vi "Open Sequence File.vi"(0 "Engine in":T3, 1 "Load Options (Default)":T2={"Use Search Dirs? (T)"=TRUE, "Conflict as Error? (T)"=TRUE, "Check Station Model? (F)"=FALSE, "Preload Modules? (T)"=TRUE, "Skip Load Callback? (F)"=FALSE, "Reload if Loaded? (F)"=FALSE}, 5 "File Path":path, 9 "Current Seq File (None)":T1, 11 "error in (no error)":errorcluster) -> (4 "Session Handle out":T3, 6 "SequenceFile":T1, 15 "error out":errorcluster)   [LabVIEW 2020, in "TSS.lvlib" / "Engine.lvclass"]
uses:
  Engine.lvclass
  Typedefs/Session Handle.ctl
  SequenceFile/Typedefs/Session Handle.ctl
  SequenceFile/SequenceFile.lvclass
  Data Types/File Load Options.ctl
  Open Sequence File Event Data.ctl
  Session Notification.ctl
  Engine.lvclass/Engine.ctl
  TSS.lvlib
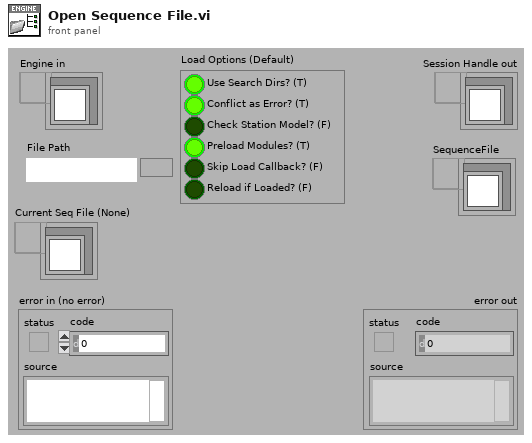
[diagram p1: front panel]
types:
  T1 = typedef "TSS.lvlib/SequenceFile.lvclass/Session Handle.ctl" = refnum<data-value>
  T2 = typedef "TSS.lvlib/File Load Options.ctl" = cluster{"Use Search Dirs? (T)":bool, "Conflict as Error? (T)":bool, "Check Station Model? (F)":bool, "Preload Modules? (T)":bool, "Skip Load Callback? (F)":bool, "Reload if Loaded? (F)":bool}
  T3 = typedef "TSS.lvlib/Engine.lvclass/Session Handle.ctl" = refnum<data-value>
  T4 = typedef "TSS.lvlib/Engine.lvclass/Session Notification.ctl" = cluster{"Session":refnum<data-value>, "Error":errorcluster}
  T5 = typedef "TSS.lvlib/Engine.lvclass/Open Sequence File Event Data.ctl" = cluster{"File Path":path, "Load Options":T2, "Current Seq File (None)":T1, "Session Notifier":refnum<notifier>, "Engine":refnum<data-value>}
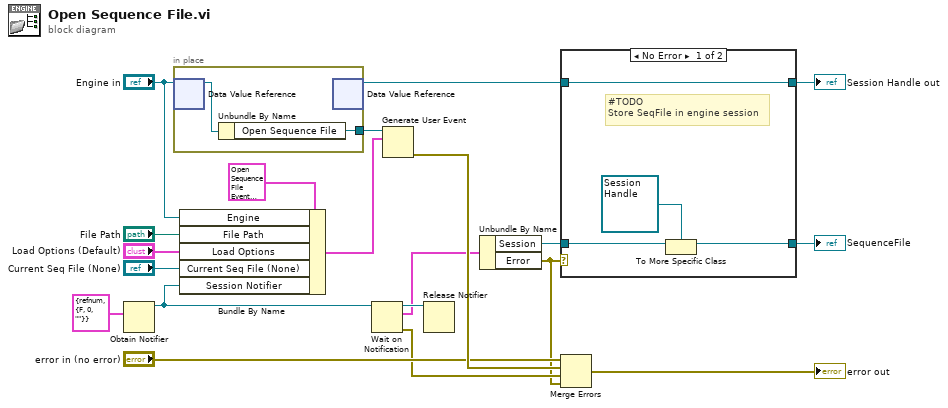
[diagram p0: block diagram]
diagram:
  n1 = Obtain Notifier(notification data type=T4 {"Session"=refnum, "Error"={"status"=FALSE, "code"=0, "source"=""}} ("Session Notification")) -> (notifier out=w11:refnum<notifier>)  [unwired: 3 in, 2 out]
  n2 = in-place {
    in-place-border: [w21] -> w13
    n3 = in-place-dvr #1("Engine in") -> (w22:refnum<class "Engine.lvclass">)  [unwired: 1 out]
    n4 = Unbundle By Name(w22) -> ("Open Sequence File"=w21:refnum<user-event>)
    n5 = in-place-dvr #1() -> (w3:T3)  [unwired: 1 in, 1 out]
  }
  n6 = Bundle By Name(cluster=T5 {"File Path"=path "", "Load Options"={"Use Search Dirs? (T)"=FALSE, "Conflict as Error? (T)"=FALSE, "Check Station Model? (F)"=FALSE, "Preload Modules? (T)"=FALSE, "Skip Load Callback? (F)"=FALSE, "Reload if Loaded? (F)"=FALSE}, "Current Seq File (None)"=refnum, "Session Notifier"=refnum, "Engine"=refnum} ("Open Sequence File Event Data"), "Engine"="Engine in", "File Path"="File Path", "Load Options"="Load Options (Default)", "Current Seq File (None)"="Current Seq File (None)", "Session Notifier"=w11) -> (w12:T5)
  n7 = Wait on Notification(notifier=w11) -> (notifier out=w10:refnum<notifier>, notification=w7:T4, error out=w9:errorcluster)  [unwired: 3 in, 1 out]
  n8 = Generate User Event(user event=w13, event data cluster=w12) -> (error out=w20:errorcluster)  [unwired: 2 in, 1 out]
  n9 = Release Notifier(notifier=w10) -> ()  [unwired: 2 in, 3 out]
  n10 = Unbundle By Name(w7) -> ("Session"=w5:refnum<data-value>, "Error"=w6:errorcluster)
  n11 = case shown="No Error" w6 {
    tunnel: w5 -> [w26 _]
    tunnel: [w24 _] -> w4
    tunnel: w3 -> [w23 w27]
    tunnel: [w23 w27] -> w2
    frame No Error {
      # "#TODO\nStore SeqFile in engine session"
      n12 = To More Specific Class(target class=T1 refnum ("SequenceFile"), reference=w26) -> (specific class reference=w24:T1)  [unwired: 1 in, 1 out]
    }
    frame Error {
    }
  }
  "Session Handle out" <- w2
  "SequenceFile" <- w4
  n13 = Merge Errors("error in (no error)", w20, w9, w6) -> (→"error out":errorcluster)
